vi "mes~产品出站.vi"(8 "error in (no error)":errorcluster caption="错误输入（无错误）", 11 "测试结果":string caption="测试结果:") -> (0 "error out":errorcluster caption="错误输出", 1 "ErrorMessage":string, 2 "出站成功":bool)   [LabVIEW 2015]
uses:
  Global.vi
  ctl/SendOutStationCommon.ctl
  ctl/ReceiveOutStationCommon.ctl
panel:
  in  "Headers":string[][](array[string])=[["Content-Type", "text/xml;charset=UTF-8"], ["SOAPAction", "\"http://tempuri.org/IOutStationServiceImpl/outStationService\""], ["Connection", "Keep-Alive"], ["User-Agent", "Apache-HttpClient/4.1.1 (java 1.5)"]]
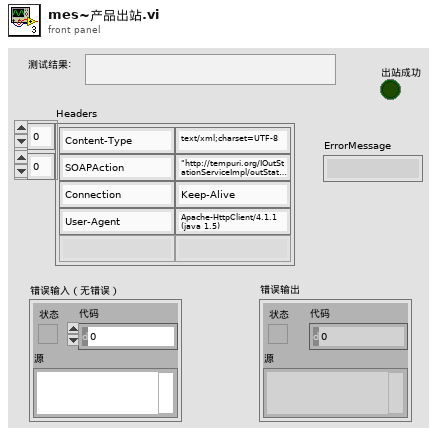
[diagram p1: front panel]
types:
  T1 = typedef "SendOutStationCommon.ctl" = cluster{"#attributes":cluster{"xmlns:soapenv":string, "xmlns:tem":string, "xmlns:cal":string}, "soapenv:Header":string, "soapenv:Body":cluster{"tem:outStationService":cluster{"tem:model":cluster{"cal:completeQty":string, "cal:equipNum":string, "cal:identiftyList":cluster{"cal:OutStationVO1":cluster{"cal:identification":string, "cal:qualityStatus":string}[]}, "cal:productType":string, "cal:siteCode":string, "cal:testOrderNum":string}}}}
  T2 = cluster{"接口地址(URL)":string, "权限校验":string, "产品进站":string, "参数采集":string, "产品出站":string, "设备状态":string, "设备编号(equipNum)":string, "站点名称(siteCode)":string, "生产类型(productType)":string, "试验单号(testOrderNum)":string}
  T3 = typedef "ReceiveOutStationCommon.ctl" = cluster{"#attributes":cluster{"xmlns:s":string}, "s:Body":cluster{"outStationServiceResponse":cluster{"#attributes":cluster{"xmlns":string}, "outStationServiceResult":cluster{"#attributes":cluster{"xmlns:a":string, "xmlns:i":string}, "a:ErrorCode":string, "a:ErrorMessage":string, "a:Success":string}}}}
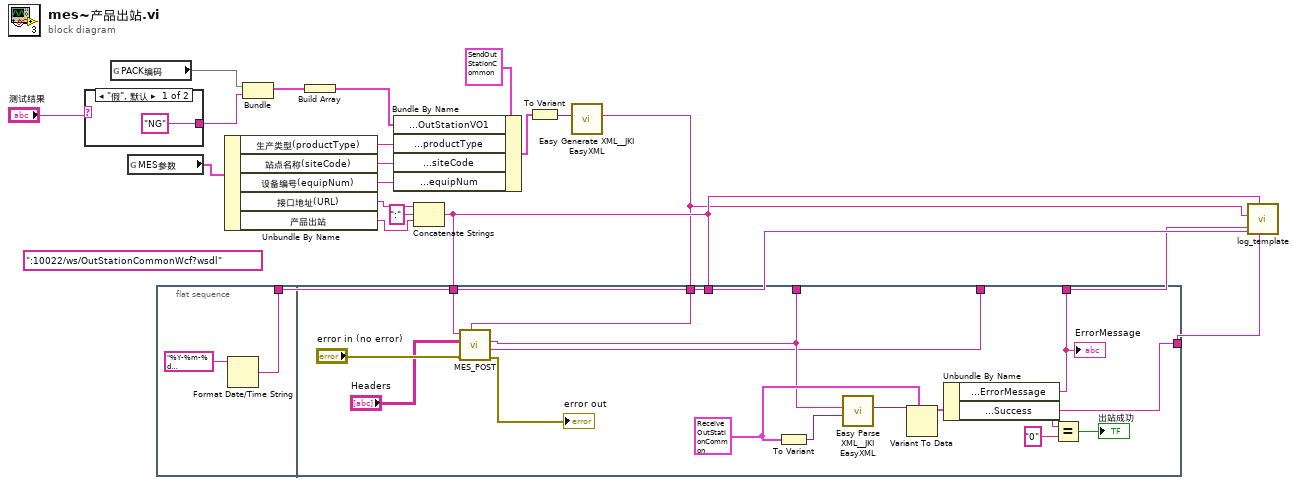
[diagram p0: block diagram]
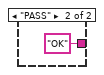
[diagram p2: hidden frame]
diagram:
  (unwired) ":10022/ws/OutStationCommonWcf?wsdl"
  n1 = case shown="\"假\", 默认" "测试结果" {
    tunnel: ["NG" "OK"] -> w8
    frame "假", Default {
    }
    frame "PASS" {
    }
  }
  n2 = global read "Global.vi" "PACK编码"() -> (w13)
  n3 = global read "Global.vi" "MES参数"() -> (w16:T2)
  n4 = flat-sequence {
    tunnel: [w23] -> w3
    tunnel: w5 -> [_]
    tunnel: w4 -> [w30]
    tunnel: [w29] -> _
    tunnel: w5 -> [w31]
    tunnel: [w28] -> _
    tunnel: [w26] -> w1
    tunnel: [w25] -> w2
    frame #0 {
      n5 = Format Date/Time String(time format string (%c)="%Y-%m-%d %H:%M:%S%3u-->" ("EndTime")) -> (date/time string=w23:string)  [unwired: 2 in]
    }
    frame #1 {
      w34 = T3 {"#attributes"={"xmlns:s"="http://schemas.xmlsoap.org/soap/envelope/"}, "s:Body"={"outStationServiceResponse"={"#attributes"={"xmlns"="http://tempuri.org/"}, "outStationServiceResult"={"#attributes"={"xmlns:a"="http://schemas.datacontract.org/2004/07/EdgeUtility", "xmlns:i"="http://www.w3.org/2001/XMLSchema-instance"}, "a:ErrorCode"="", "a:ErrorMessage"="", "a:Success"=""}}}} ("s:Envelope")
      n6 = call "MES_POST.vi"("DATA"=w30, "错误输入（无错误）"="error in (no error)", 10:"Headers", "URL"=w31) -> ("错误输出"=→"error out":errorcluster, "headers"=w28:string, "body"=w29:string)  [unwired: 5 in]
      n7 = To Variant(anything=w34) -> (Variant=w39:variant)
      n8 = call <vilib>:"Easy Parse XML__JKI EasyXML.vi"("LabVIEW Data (Type)"=w39, "XML String"=w29) -> ("LabVIEW Data"=w38:variant)  [unwired: 8 in, 1 out]
      n9 = Variant To Data(type=w34, Variant=w38) -> (data=w37:T3)  [unwired: 1 in, 1 out]
      n10 = Unbundle By Name(w37) -> ("s:Body.outStationServiceResponse.outStationServiceResult.a:ErrorMessage"=w26:string, "s:Body.outStationServiceResponse.outStationServiceResult.a:Success"=w25:string)
      "ErrorMessage" <- w26
      n11 = Equal?(x=w25, y="0") -> (x = y?=→"出站成功":bool)
    }
  }
  n12 = Unbundle By Name(w16) -> ("生产类型(productType)"=w14:string, "站点名称(siteCode)"=w17:string, "设备编号(equipNum)"=w18:string, "接口地址(URL)"=w15:string, "产品出站"=w6:string)
  n13 = Bundle("PACK编码"=w13, w8) -> (w12:cluster{"PACK编码":void, string})  [unwired: 1 in]
  n14 = Build Array(w12) -> (w11:cluster{"PACK编码":void, string}[])
  n15 = Bundle By Name(cluster=T1 {"#attributes"={"xmlns:soapenv"="http://schemas.xmlsoap.org/soap/envelope/", "xmlns:tem"="http://tempuri.org/", "xmlns:cal"="http://schemas.datacontract.org/2004/07/CalbOutStationCommonService"}, "soapenv:Header"="", "soapenv:Body"={"tem:outStationService"={"tem:model"={"cal:completeQty"="", "cal:equipNum"="", "cal:identiftyList"={"cal:OutStationVO1"=[]}, "cal:productType"="", "cal:siteCode"="", "cal:testOrderNum"=""}}}} ("soapenv:Envelope"), "soapenv:Body.tem:outStationService.tem:model.cal:identiftyList.cal:OutStationVO1"=w11, "soapenv:Body.tem:outStationService.tem:model.cal:productType"=w14, "soapenv:Body.tem:outStationService.tem:model.cal:siteCode"=w17, "soapenv:Body.tem:outStationService.tem:model.cal:equipNum"=w18) -> (w20:T1)
  n16 = Concatenate Strings(w15, ":" ("字符串"), w6) -> (w5:string)
  n17 = To Variant(anything=w20) -> (Variant=w19:variant)
  n18 = call <vilib>:"Easy Generate XML__JKI EasyXML.vi"("LabVIEW Data"=w19) -> ("XML String"=w4:string)  [unwired: 9 in, 1 out]
  n19 = call "log_template.vi"(4:w1, 6:w2, 7:w5, 8:w3, 10:w4) -> ()  [unwired: 7 in]
